vi "Read DAQmx Device Name.vi"(8 "error in (no error)":errorcluster, 11 "National Instrument USB-6501 in":refnum<class "National Instrument USB-6501.lvclass">) -> (0 "error out":errorcluster, 2 "DAQmx Device Name":tag, 3 "National Instrument USB-6501 out":refnum<class "National Instrument USB-6501.lvclass">)   [LabVIEW 2014, in "Generic Data Acquisition.lvlib" / "National Instrument USB-6501.lvlib" / "National Instrument USB-6501.lvclass"]
uses:
  National Instrument USB-6501.lvclass
  National Instrument USB-6501.lvclass/National Instrument USB-6501.ctl
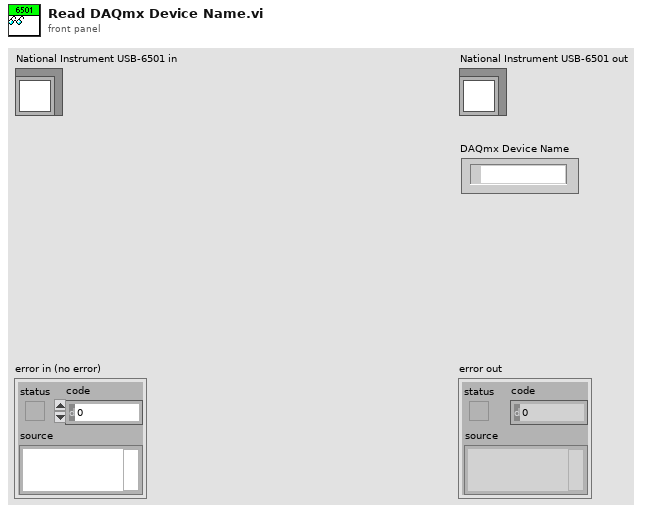
[diagram p1: front panel]
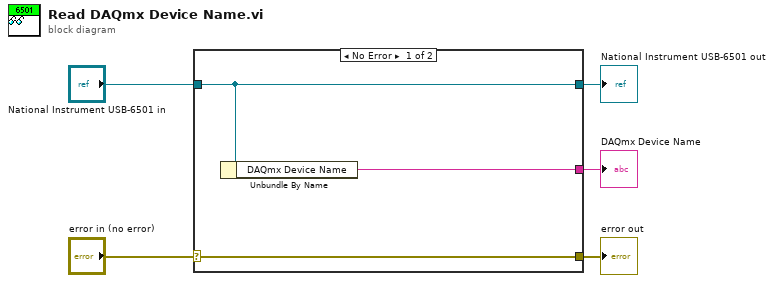
[diagram p0: block diagram]
diagram:
  n1 = case shown="No Error" "error in (no error)" {
    selector: "error in (no error)" -> [w8 w9]
    tunnel: [w8 w9] -> w4
    tunnel: [w7 w10] -> w2
    tunnel: "National Instrument USB-6501 in" -> [w7 w10]
    tunnel: [w6 _] -> w1
    frame No Error {
      n2 = Unbundle By Name(w7) -> ("DAQmx Device Name"=w6:tag)
    }
    frame Error {
    }
  }
  "error out" <- w4
  "National Instrument USB-6501 out" <- w2
  "DAQmx Device Name" <- w1
